vi "Close Galil IO.vi"(3 "Error In":errorcluster, 4 "Command Input":string, 5 "Reference In":refnum<k7>) -> (0 "Error Out":errorcluster, 1 "Command Output":string)   [LabVIEW 2011]
uses:
  _GlobalVariables&Libraries/ATV Program Global Variables.vi
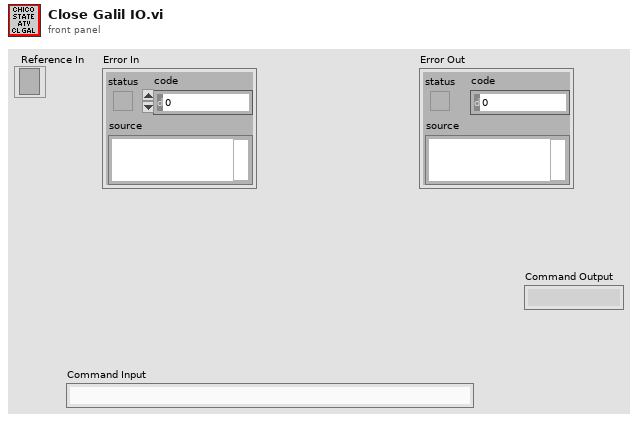
[diagram p1: front panel]
types:
  T1 = cluster{"Drive Value Output String":string, "Steer Value Output String":string, "Error Out":errorcluster, "Initial Encoder Counts":string, "Disable Galil Terminal":bool, "Command Input":string}
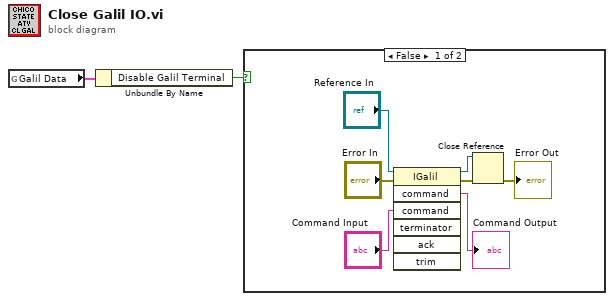
[diagram p0: block diagram]
diagram:
  n1 = global read "ATV Program Global Variables.vi" "Galil Data"() -> (w2:T1)
  n2 = Unbundle By Name(w2) -> ("Disable Galil Terminal"=w1:bool)
  n3 = case shown="False" w1 {
    frame False {
      n4 = invoke class="IGalil" method="command"(reference="Reference In", error in="Error In", "command"="Command Input") -> (reference out=w5:refnum<k7>, error out=w4:errorcluster, "command"=→"Command Output":string)  [unwired: 4 in, 4 out]
      n5 = Close Reference(reference=w5, error in (no error)=w4) -> (error out=→"Error Out":errorcluster)
    }
    frame True {
    }
  }
